vi "Get Notifier Ref.vi"(8 "error in (no error)":errorcluster, 11 "CVT_Boolean in":refnum<class "CVT_Boolean.lvclass">) -> (0 "error out":errorcluster, 2 "notifier out":refnum<notifier>, 3 "CVT_Boolean out":refnum<class "CVT_Boolean.lvclass">)   [LabVIEW 2024, in "Current Value Table.lvlib" / "CVT_Boolean.lvclass"]
uses:
  CVT_Boolean.lvclass
  CVT_Boolean.lvclass/CVT_Boolean.ctl
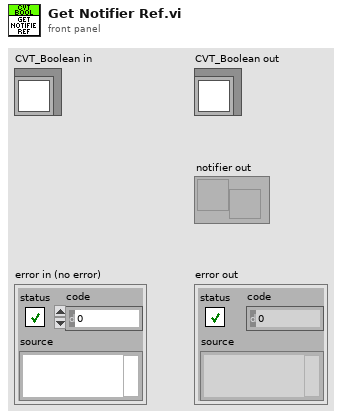
[diagram p1: front panel]
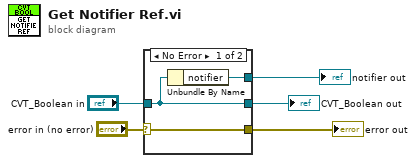
[diagram p0: block diagram]
diagram:
  n1 = case shown="No Error" "error in (no error)" {
    selector: "error in (no error)" -> [w8 w10]
    tunnel: [w8 w10] -> w4
    tunnel: [w7 w9] -> w2
    tunnel: "CVT_Boolean in" -> [w7 w9]
    tunnel: [w6 _] -> w1
    frame No Error {
      n2 = Unbundle By Name(w7) -> ("notifier"=w6:refnum<notifier>)
    }
    frame Error {
    }
  }
  "error out" <- w4
  "CVT_Boolean out" <- w2
  "notifier out" <- w1
